vi "Find Latest Fine Mask File.vi"(8 "error in":errorcluster, 9 "RawData Save Path":path=path "C:/Users/Flash/Desktop/Data/Detector test data", 10 "Device Name":string="Diode_Open_5_100", 11 "Wafer Name":string="A-3348-2-A") -> (0 "Error Out":errorcluster, 3 "Mask File Fine":path=path "C:/Users/Flash/Desktop/Mask Files/SL066 Detector/SL066_D5_20_align on D3000.csv")   [LabVIEW 2012]
panel:
  out "element":cluster{"last mod":timestamp, i32}
  out "Array":timestamp[](array[timestamp])
  out "filenames":string[](array[string])
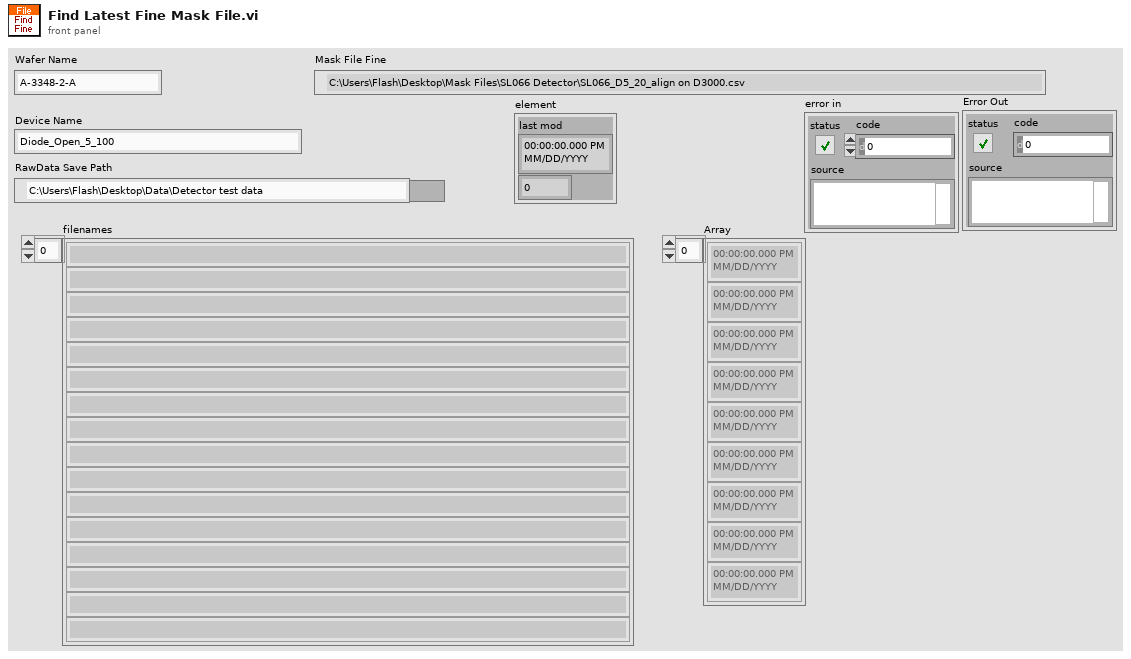
[diagram p1: front panel]
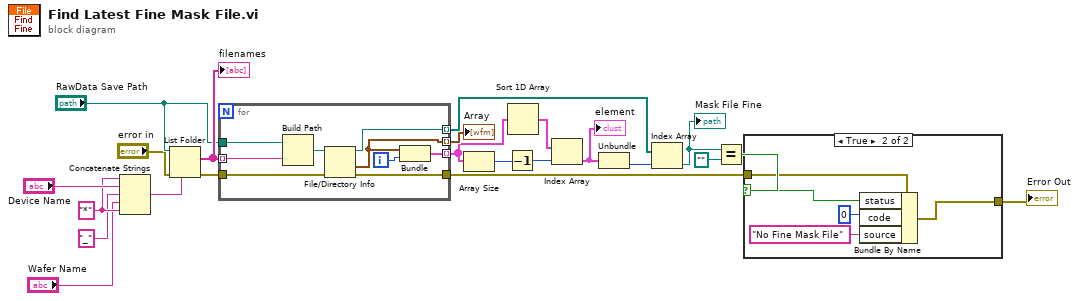
[diagram p0: block diagram]
diagram:
  w20 = "*" ("string")
  n1 = Concatenate Strings(w20, "Device Name", "_" ("string"), "Wafer Name", w20) -> (w19:string)
  n2 = List Folder(path="RawData Save Path", pattern=w19, error in="error in") -> (filenames=w22:string[], error out=w4:errorcluster)  [unwired: 1 in, 2 out]
  "filenames" <- w22
  n3 = for {
    tunnel: w22 -> [w30] mode=indexing
    tunnel: "RawData Save Path" -> [w31]
    tunnel: [w27] -> w15 mode=indexing
    tunnel: [w28] -> w8 mode=indexing
    tunnel: [w25] -> w13 mode=indexing
    tunnel: w4 -> [w24]
    tunnel: [w23] -> w3
    i -> [w26]
    n4 = Build Path(base path=w31, name or relative path=w30) -> (appended path=w29:path)
    n5 = File/Directory Info(path=w29, error in=w24) -> (path out=w28:path, last mod=w27:timestamp, error out=w23:errorcluster)  [unwired: 4 out]
    n6 = Bundle("last mod"=w27, w26) -> (w25:cluster{"last mod":timestamp, i32})  [unwired: 1 in]
  }
  "Array" <- w15
  n7 = Array Size(array=w13) -> (size(s)=w12:i32)
  n8 = Decrement(x=w12) -> (x-1=w11:i32)
  n9 = Sort 1D Array(array=w13) -> (sorted array=w14:cluster{"last mod":timestamp, i32}[])
  n10 = Index Array(array=w14, index=w11) -> (element=w10:cluster{"last mod":timestamp, i32})
  "element" <- w10
  n11 = Unbundle(w10) -> (w9:i32)  [unwired: 1 out]
  n12 = Index Array(array=w8, index=w9) -> (element=w7:path)
  "Mask File Fine" <- w7
  n13 = Equal?(x=w7, y=path "") -> (x = y?=w2:bool)
  n14 = case shown="True" w2 {
    selector: w2 -> [_ w35]
    tunnel: w3 -> [w32 w37]
    tunnel: [w32 w36] -> w1
    frame False {
    }
    frame True {
      n15 = Bundle By Name(cluster=w37, "status"=w35, "code"=0, "source"="No Fine Mask File") -> (w36:errorcluster)
    }
  }
  "Error Out" <- w1
